vi "未命名 1 (子VI).vi"(0 "标准体积 4":dbl, 1 "标准体积 3":dbl, 2 "标准体积输入":dbl, 3 "标准体积 1":dbl, 5 "标准体积 5":dbl, 7 "实际体积 1":dbl, 9 "实际体积输入":dbl, 12 "实际体积 3":dbl, 13 "实际体积 4":dbl, 14 "实际体积 5":dbl) -> (4 "拟合方程":string, 6 "r^2":dbl format="%_6g", 8 "B":dbl caption="截距", 10 "K":dbl caption="斜率")   [LabVIEW 2016]
uses:
  <vilib>/Analysis/6fits.llb/Curve Fitting Criteria.ctl
  <vilib>/Analysis/NI_AALPro.lvlib
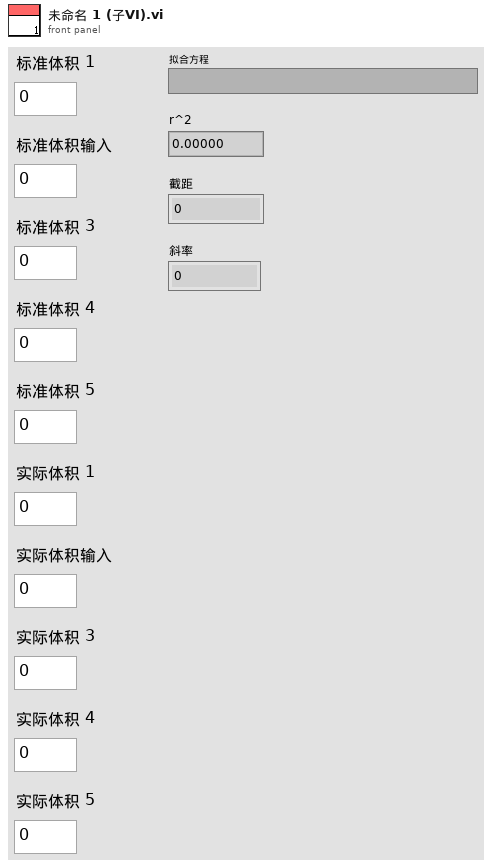
[diagram p1: front panel]
types:
  T1 = typedef "NI_AALPro.lvlib/Curve Fitting Criteria.ctl" = u16
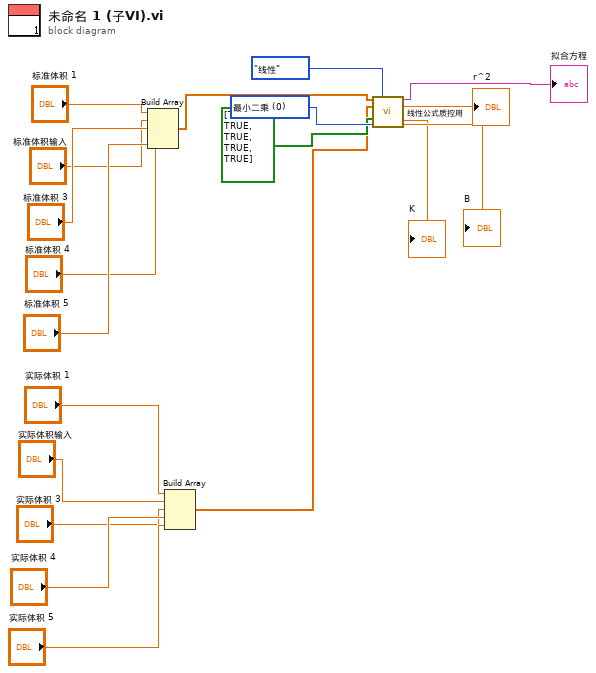
[diagram p0: block diagram]
diagram:
  w14 = T1 0 items=["最小二乘", "最小绝对残差", "Bisquare"] ("method")
  n1 = Build Array("标准体积 1", "标准体积输入", "标准体积 3", "标准体积 4", "标准体积 5") -> (w11:dbl[])
  n2 = Build Array("实际体积 1", "实际体积输入", "实际体积 3", "实际体积 4", "实际体积 5") -> (w12:dbl[])
  n3 = call "线性公式质控用.vi"("标液浓度"=w11, "模型"=enum32{"线性", "多项式"}."线性", "监测浓度"=w12, "启用"=bool[] [TRUE, TRUE, TRUE, TRUE, TRUE], "method"=w14) -> ("拟合方程"=→"拟合方程":string, "r^2"=→"r^2":dbl, "slope"=→"K":dbl, "intercept"=→"B":dbl)  [unwired: 6 in, 1 out]
